vi "CPP-ZeroChannels.vi"(1 "SecondsToAverage":dbl, 2 "ADAM Ch Names":string[](array[string])) -> (0 "Seconds since 1 Jan 1904":dbl)   [LabVIEW 2015]
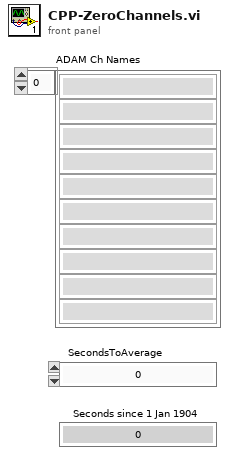
[diagram p1: front panel]
types:
  T1 = typedef "Ch_description_ADAM.ctl" = cluster{"Ch Name":string, "Type":T2, "Function":T3, "Ch State":T4, "Calibration type":T5, "A":dbl, "B":dbl, "C":dbl, "D":dbl, "Comments":string, "Address":T6, "String":string, "Duty":u16}
  T2 = typedef "Module_type_ADAM.ctl" = string
  T3 = typedef "Function_ADAM.ctl" = enum16{"Analogue Input", "Digital Input", "Event counter", "Event rate", "Analogue Output", "Digital Output", "Relay Output"}
  T4 = typedef "Channel_State.ctl" = enum16{"On", "Off", "Always On", "Always Off"}
  T5 = typedef "Calib_type_ADAM.ctl" = enum16{"Raw", "Bx + A", "Cx^2 + Bx + A", "Dx^3 + Cx^2 + Bx + A", "In Band", "Hi-Tec Q", "Hi-Tec M_dot", "Text"}
  T6 = typedef "Address.ctl" = cluster{"Main":i32, "Ch.":i32, "Sub":i32, "Port Name":string}
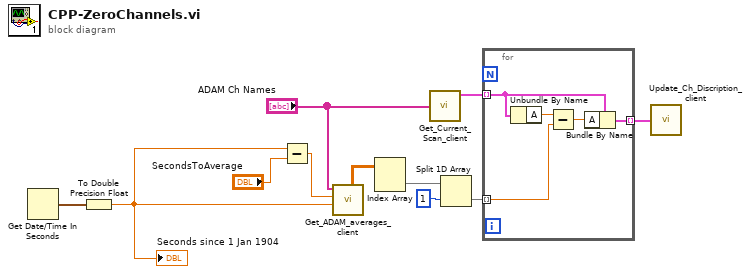
[diagram p0: block diagram]
diagram:
  n1 = Get Date/Time In Seconds() -> (seconds since 1Jan1904=w11:timestamp)
  n2 = To Double Precision Float(number=w11) -> (double precision float=w2:dbl)
  "Seconds since 1 Jan 1904" <- w2
  n3 = Subtract(x=w2, y="SecondsToAverage") -> (x-y=w3:dbl)
  n4 = call "Get_ADAM_averages_client.vi"("End time"=w2, "Start time"=w3, "ADAM Ch Names"="ADAM Ch Names") -> ("DBL values"=w8:dbl[][])  [unwired: 4 in, 4 out]
  n5 = Index Array(array=w8) -> (element=w7:dbl[])  [unwired: 2 in]
  n6 = call "Get_Current_Scan_client.vi"("ADAM Ch Names"="ADAM Ch Names") -> ("Ch Description Array"=w9:T1[])  [unwired: 3 out]
  n7 = Split 1D Array(array=w7, index=1) -> (second subarray=w6:dbl[])  [unwired: 1 out]
  n8 = for {
    tunnel: w9 -> [w14] mode=indexing
    tunnel: w6 -> [w15] mode=indexing
    tunnel: [w12] -> w4 mode=indexing
    n9 = Unbundle By Name(w14) -> ("A"=w16:dbl)
    n10 = Subtract(x=w16, y=w15) -> (x-y=w13:dbl)
    n11 = Bundle By Name(cluster=w14, "A"=w13) -> (w12:T1)
  }
  n12 = call "Update_Ch_Discription_client.vi"("Channels to update In"=w4) -> ()  [unwired: 1 out]
